vi "Cal Inst current voltage waveforms.vi"(8 "error in (no error)":errorcluster, 11 "VISA resource name":refnum<visa-resource-name>) -> (0 "error out":errorcluster, 2 "Waveform Graph":waveform(sgl)[](graph), 3 "VISA resource name out":refnum<visa-resource-name>)   [LabVIEW 2013]
uses:
  Libraries/California Instruments iX Series/California Instruments iX Series.lvlib
  Cal Inst Acquisition.lvlib
panel:
  in  "ACQ length (1-10)":i32=1
  out "return count 3":u32
  out "Number of Bytes at Port":u32
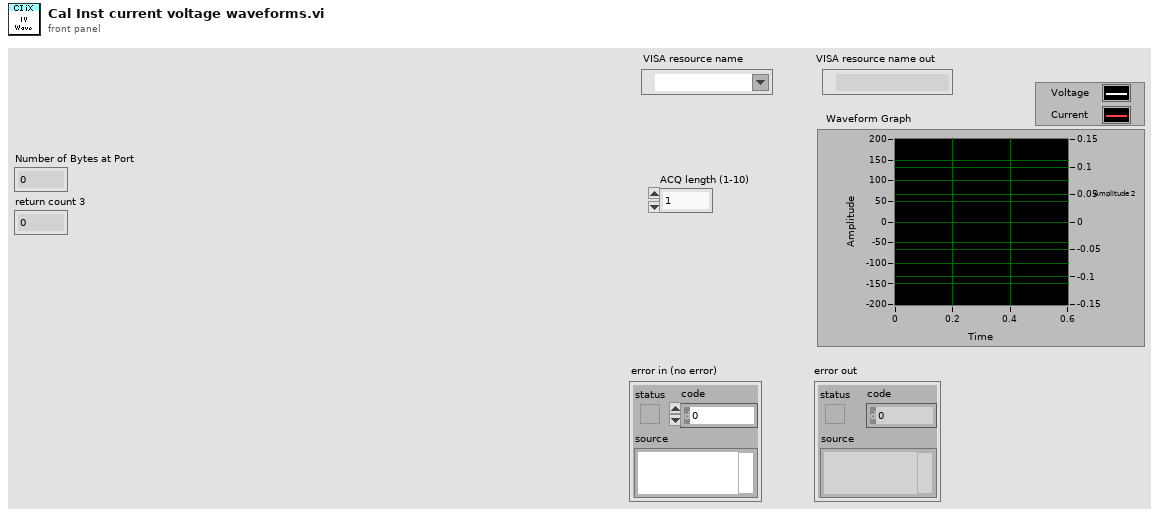
[diagram p1: front panel]
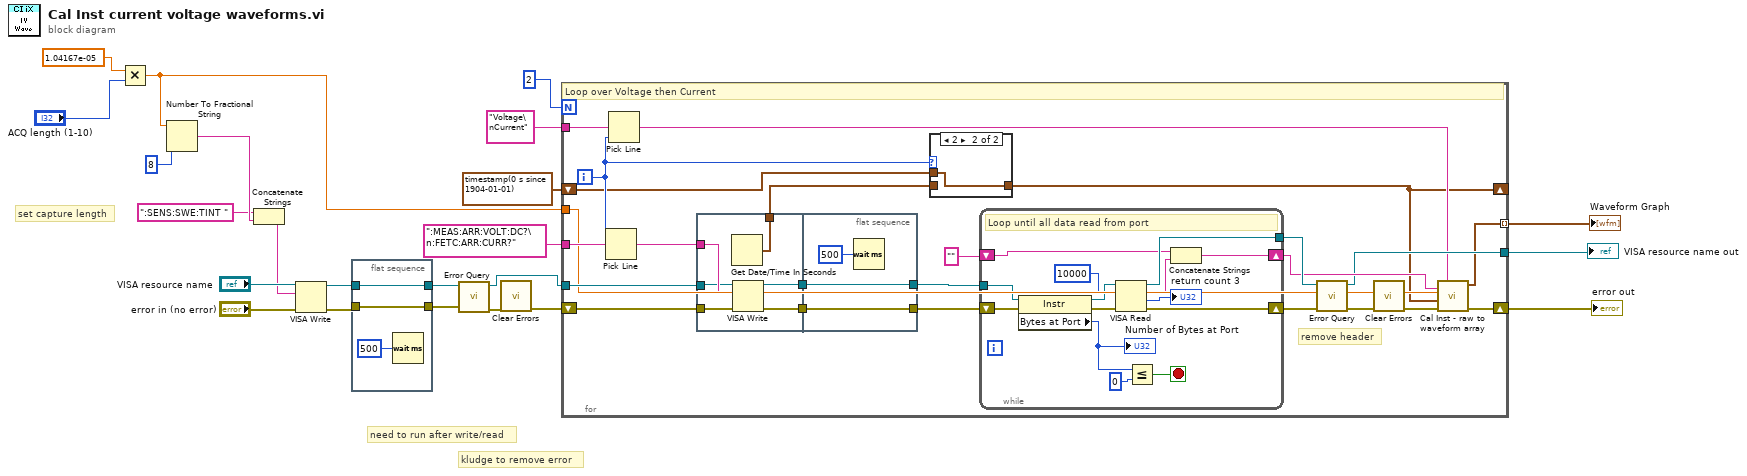
[diagram p0: block diagram]
diagram:
  # "kludge to remove error"
  # "need to run after write/read"
  # "set capture length"
  n1 = Multiply(x=1.04167e-05, y="ACQ length (1-10)") -> (x*y=w2:dbl)
  n2 = Number To Fractional String(number=w2, precision (6)=i16 8) -> (F-format string=w17:string)  [unwired: 2 in]
  n3 = Concatenate Strings(":SENS:SWE:TINT " ("multi-line string"), w17) -> (w3:string)
  n4 = VISA Write(VISA resource name="VISA resource name", write buffer=w3, error in (no error)="error in (no error)") -> (VISA resource name out=w11:refnum<visa-resource-name>, error out=w12:errorcluster)  [unwired: 1 out]
  n5 = flat-sequence {
    tunnel: w12 -> [w25]
    tunnel: [w25] -> w6
    tunnel: w11 -> [w24]
    tunnel: [w24] -> w5
    frame #0 {
      n6 = Wait (ms)(milliseconds to wait=u32 500) -> ()  [unwired: 1 out]
    }
  }
  n7 = call "Error Query.vi"("error in (no error)"=w6, "VISA resource name"=w5) -> ("error out"=w15:errorcluster, "VISA resource name out"=w14:refnum<visa-resource-name>)  [unwired: 6 in, 2 out]
  n8 = call <vilib>:"Clear Errors.vi"("error in (no error)"=w15) -> ("error out"=w13:errorcluster)  [unwired: 6 in]
  n9 = for {
    N: 2 -> [_]
    tunnel: ":MEAS:ARR:VOLT:DC?\n:FETC:ARR:CURR?" ("multi-line string") -> [w46]
    shift-right: [w32] -> w21
    shift-left: w13 -> [w39]
    tunnel: [w44] -> w20
    tunnel: w14 -> [w42]
    tunnel: "Voltage\nCurrent" ("multi-line string") -> [w36]
    tunnel: [w34] -> w18 mode=indexing
    tunnel: w2 -> [w31]
    shift-right: [w28] -> _
    shift-left: timestamp(0 s since 1904-01-01) ("seconds since 1Jan1904") -> [w27]
    i -> [w29]
    # "remove header"
    # "Loop over Voltage then Current"
    n10 = Pick Line(multi-line string=w46, line index=w29) -> (output string=w43:string)  [unwired: 1 in]
    n11 = Pick Line(multi-line string=w36, line index=w29) -> (output string=w35:string)  [unwired: 1 in]
    n12 = flat-sequence {
      tunnel: w43 -> [w72]
      tunnel: w42 -> [w71]
      tunnel: [w70] -> w41
      tunnel: [w69] -> w30
      tunnel: w39 -> [w68]
      tunnel: [w67] -> w38
      tunnel: w41 -> [w74]
      tunnel: [w74] -> w40
      tunnel: [w73] -> w37
      tunnel: w38 -> [w73]
      frame #0 {
        n13 = Get Date/Time In Seconds() -> (seconds since 1Jan1904=w69:timestamp)
        n14 = VISA Write(VISA resource name=w71, write buffer=w72, error in (no error)=w68) -> (VISA resource name out=w70:refnum<visa-resource-name>, error out=w67:errorcluster)  [unwired: 1 out]
      }
      frame #1 {
        n15 = Wait (ms)(milliseconds to wait=u32 500) -> ()  [unwired: 1 out]
      }
    }
    n16 = case shown="2" w29 {
      tunnel: w30 -> [w51 _]
      tunnel: [w51 w52] -> w28
      tunnel: w27 -> [_ w52]
      frame 1, Default {
      }
      frame 2 {
      }
    }
    n17 = while {
      tunnel: [w65] -> w48
      shift-right: [w54] -> w45
      shift-left: "" -> [w63]
      shift-right: [w58] -> w49
      shift-left: w37 -> [w59]
      tunnel: w40 -> [w53]
      stop <- w55 stop-if-true
      # "Loop until all data read from port"
      n18 = property class="Instr"(reference=w53, error in=w59) -> (reference out=w61:refnum<visa-resource-name>, error out=w60:errorcluster, "Bytes at Port"=w57:u32)
      "Number of Bytes at Port" <- w57
      n19 = VISA Read(VISA resource name=w61, byte count=u32 10000, error in (no error)=w60) -> (VISA resource name out=w65:refnum<visa-resource-name>, read buffer=w62:string, return count=→"return count 3":u32, error out=w58:errorcluster)
      n20 = Less Or Equal?(x=w57, y=u32 0) -> (x <= y?=w55:bool)
      n21 = Concatenate Strings(w63, w62) -> (w54:string)
    }
    n22 = call "Error Query.vi"("error in (no error)"=w49, "VISA resource name"=w48) -> ("error out"=w50:errorcluster, "VISA resource name out"=w44:refnum<visa-resource-name>)  [unwired: 6 in, 2 out]
    n23 = call <vilib>:"Clear Errors.vi"("error in (no error)"=w50) -> ("error out"=w33:errorcluster)  [unwired: 6 in]
    n24 = call "Cal Inst - raw to waveform array.vi"("String"=w45, "error in (no error)"=w33, "seconds since 1Jan1904"=w28, "Numeric"=w31, "output string"=w35) -> ("error out"=w32:errorcluster, "Waveform"=w34:waveform(sgl))  [unwired: 5 in]
  }
  "Waveform Graph" <- w18
  "error out" <- w21
  "VISA resource name out" <- w20
